vi "DrawBuoy.vi"(1 "(xr,yr) old":cluster{"x robot":dbl, "y robot":dbl}, 2 "(xr,yr) new":cluster{"x robot":dbl, "y robot":dbl}, 3 "2D Picture":picture) -> (0 "new picture":picture)   [LabVIEW 2012]
doc: "Draws a magenta circle at the curretn (x,y) coordinates of the Robot in the current mission definition file.\nInputs:\nPicture to draw on\nCluster X\n y coordinates of robot\nOutput:\nmodified picture"
panel:
  # "Draws a circle at the current x,y coordinates of the robot"
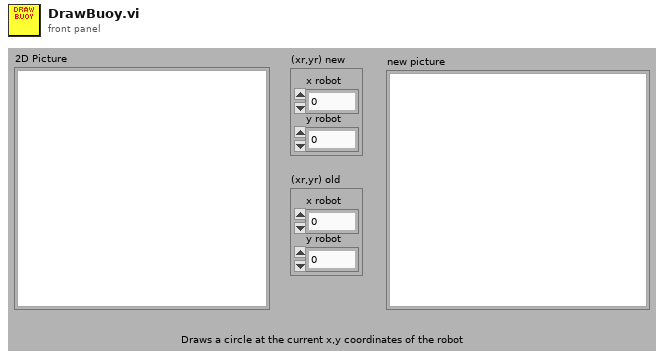
[diagram p1: front panel]
types:
  T1 = cluster{"Width":u16, "Style":enum32{"Solid", "Dash", "Dot", "DashDot", "DashDotDot"}}
  T2 = typedef "imagedata.ctl" = cluster{"image type":i32, "image depth":i32, "image":u8[], "mask":u8[], "colors":u32[], "Rectangle":cluster{"left":i16, "top":i16, "right":i16, "bottom":i16}}
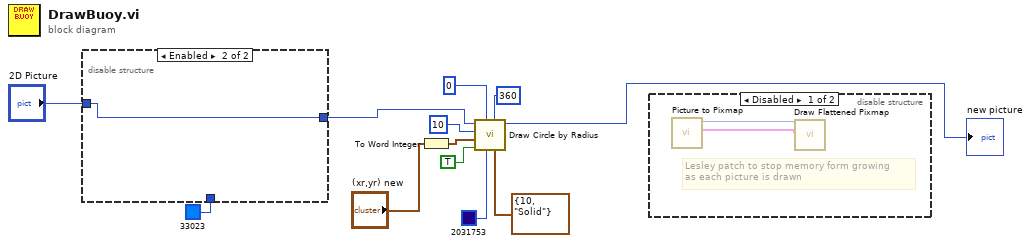
[diagram p0: block diagram]
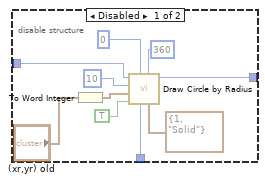
[diagram p2: hidden frame]
diagram:
  n1 = disable-structure shown="Enabled" {
    disable-tunnel: u32 33023 ("color(black)") -> [w20 _]
    disable-tunnel: "2D Picture" -> [w14 w23]
    disable-tunnel: [w13 w23] -> w1
    frame Disabled {
      n2 = To Word Integer(number="(xr,yr) old") -> (16bit integer=w16:cluster{"x robot":i16, "y robot":i16})
      n3 = call <vilib>:"Draw Circle by Radius.vi"("pen"=T1 {"Width"=1, "Style"=enum."Solid"}, "arc size(360)"=i16 360, "color(black)"=w20, "start angle(0)"=i16 0, "fill?(F)"=TRUE, "pixel center"=w16, "radius"=i16 10, "picture"=w14) -> ("new picture"=w13:picture)  [unwired: 3 in]
    }
    frame Enabled {
    }
  }
  n4 = To Word Integer(number="(xr,yr) new") -> (16bit integer=w12:cluster{"x robot":i16, "y robot":i16})
  n5 = call <vilib>:"Draw Circle by Radius.vi"("pen"=T1 {"Width"=10, "Style"=enum."Solid"}, "arc size(360)"=i16 360, "color(black)"=u32 2031753, "start angle(0)"=i16 0, "fill?(F)"=TRUE, "pixel center"=w12, "radius"=i16 10, "picture"=w1) -> ("new picture"=→"new picture":picture)  [unwired: 3 in]
  n6 = disable-structure shown="Disabled" {
    frame Disabled {
      # "Lesley patch to stop memory form growing\nas each picture is drawn"
      n7 = call <vilib>:"Picture to Pixmap.vi"() -> ("image data"=w24:T2, "new picture"=w25:picture)  [unwired: 10 in]
      n8 = call <vilib>:"Draw Flattened Pixmap.vi"("image data"=w24, "picture"=w25) -> ()  [unwired: 7 in, 1 out]
    }
    frame Enabled {
    }
  }
